vi "john read wavelength.vi"() -> ()   [LabVIEW 2012]
uses:
  Global/GPIB Numbers.vi
panel:
  out "Current WL":dbl
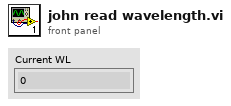
[diagram p1: front panel]
types:
  T1 = typedef "USBCCD Type Def.ctl" = cluster{"Name":string, "Unique ID":string, "Mono Unique ID":string}
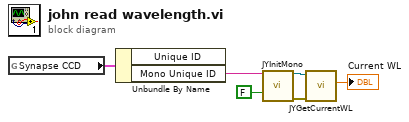
[diagram p0: block diagram]
diagram:
  n1 = global read "GPIB Numbers.vi" "Synapse CCD"() -> (w4:T1)
  n2 = Unbundle By Name(w4) -> ("Mono Unique ID"=w2:string)  [unwired: 1 out]
  n3 = call "JYInitMono.vi"("Unique ID"=w2, "Force Init"=FALSE) -> ("Mono RefNum out"=w6:refnum<k7>, "error out"=w5:errorcluster)  [unwired: 9 in, 3 out]
  n4 = call "JYGetCurrentWL.vi"("error in (no error)"=w5, "JYMONOLib.IJYMonoReqd In"=w6) -> ("Current WL"=→"Current WL":dbl)  [unwired: 6 in, 3 out]
